vi "PopulateClearModes.vi"(10 "ClearingModes":refnum<k24>, 11 "ComboBox in":refnum<vi>) -> ()   [LabVIEW 2018]
uses:
  D:/SVN/PM/sdk/AppSamples/LabVIEWSamples/trunk/Release/2018/Dependencies/PVCamNET.dll
  Dependencies/PVCamNET.dll
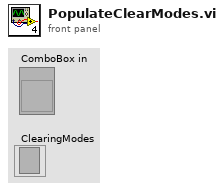
[diagram p1: front panel]
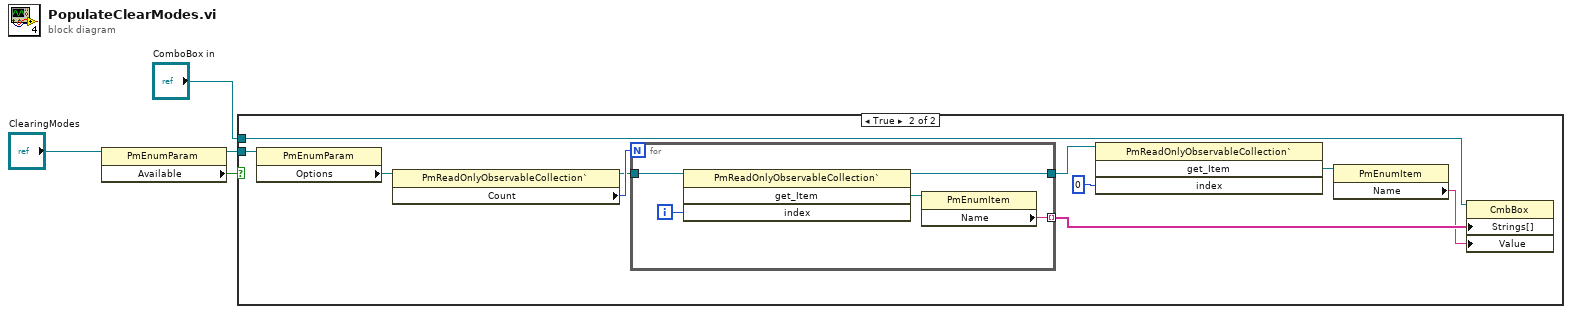
[diagram p0: block diagram]
diagram:
  n1 = property class="PmEnumParam"(reference="ClearingModes") -> (reference out=w3:refnum<k24>, "Available"=w2:bool)  [unwired: 1 in, 1 out]
  n2 = case shown="True" w2 {
    tunnel: w3 -> [_ w14]
    tunnel: "ComboBox in" -> [_ w5]
    frame False {
    }
    frame True {
      n3 = property class="PmEnumParam"(reference=w14) -> ("Options"=w13:refnum<k24>)  [unwired: 1 in, 2 out]
      n4 = property class="PmReadOnlyObservableCollection`"(reference=w13) -> (reference out=w11:refnum<k24>, "Count"=w12:i32)  [unwired: 1 in, 1 out]
      n5 = for {
        N: w12 -> [_]
        tunnel: w11 -> [w19]
        tunnel: [w16] -> w9
        tunnel: [w15] -> w10 mode=indexing
        i -> [w18]
        n6 = invoke class="PmReadOnlyObservableCollection`" method="get_Item"(reference=w19, "index"=w18) -> (reference out=w16:refnum<k24>, "get_Item"=w17:refnum<k24>)  [unwired: 2 in, 2 out]
        n7 = property class="PmEnumItem"(reference=w17) -> ("Name"=w15:string)  [unwired: 1 in, 2 out]
      }
      n8 = invoke class="PmReadOnlyObservableCollection`" method="get_Item"(reference=w9, "index"=0) -> ("get_Item"=w7:refnum<k24>)  [unwired: 2 in, 3 out]
      n9 = property class="PmEnumItem"(reference=w7) -> ("Name"=w6:string)  [unwired: 1 in, 2 out]
      n10 = property class="CmbBox"(reference=w5, "Strings[]"=w10, "Value"=w6) -> ()  [unwired: 1 in, 2 out]
    }
  }
